vi "INIT-Sequence.vi"(8 "error in (no error)":errorcluster, 9 "TDX":bool[](array[boolean]), 10 "DelayuS":i32=7, 11 "VISA resource name IN":refnum<visa-resource-name>) -> (0 "error out":errorcluster, 1 "TRANSD":u16, 2 "Tamaño Script":i32, 3 "VISA resource name OUT":refnum<visa-resource-name>)   [LabVIEW 2014, in "CAP-USB.lvlib"]
uses:
  CAP-USB.lvlib
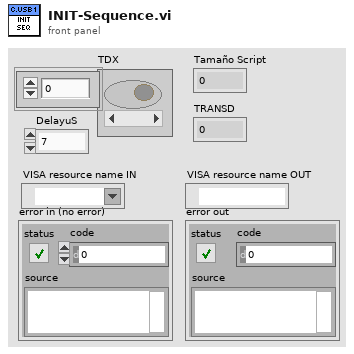
[diagram p1: front panel]
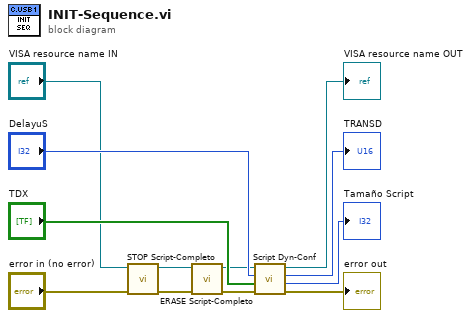
[diagram p0: block diagram]
diagram:
  n1 = call "STOP Script-Completo.vi"("error in (no error)"="error in (no error)", "VISA resource name"="VISA resource name IN") -> ("error out"=w3:errorcluster, "VISA resource name out"=w4:refnum<visa-resource-name>)  [unwired: 8 in]
  n2 = call "ERASE Script-Completo.vi"("error in (no error)"=w3, "VISA resource name"=w4) -> ("error out"=w1:errorcluster, "VISA resource name out"=w2:refnum<visa-resource-name>)  [unwired: 8 in]
  n3 = call "Script Dyn-Conf.vi"("error in (no error)"=w1, "TDX"="TDX", "DelayuS"="DelayuS", "VISA resource name IN"=w2) -> ("error out"=→"error out":errorcluster, "Tamaño Script"=→"Tamaño Script":i32, "TRANSD"=→"TRANSD":u16, "VISA resource name OUT"=→"VISA resource name OUT":refnum<visa-resource-name>)  [unwired: 2 in]
